vi "EMMA(SubVI).vi"(10 "Constante alpha":dbl, 11 "Entrada del filtro":dbl) -> (3 "x+y":dbl)   [LabVIEW 2020]
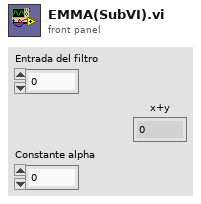
[diagram p1: front panel]
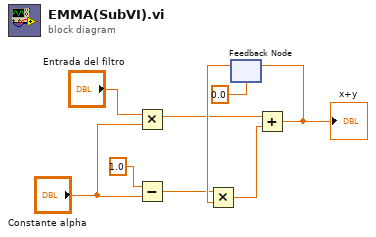
[diagram p0: block diagram]
diagram:
  n1 = Multiply(x="Entrada del filtro", y="Constante alpha") -> (x*y=w5:dbl)
  n2 = Subtract(x=1.0, y="Constante alpha") -> (x-y=w4:dbl)
  n3 = feedback #1(0.0) -> (w7:dbl)
  n4 = Multiply(x=w4, y=w7) -> (x*y=w8:dbl)
  n5 = Add(x=w5, y=w8) -> (x+y=w6:dbl)
  "x+y" <- w6
  n6 = feedback-in #1(w6) -> ()
